vi "CSV reader.vi"(9 "x":dbl, 10 "Array":string[](array[string]), 11 "Number CSV":dbl) -> ()   [LabVIEW 2014]
uses:
  <vilib>/Utility/file.llb/Read From Spreadsheet File (DBL).vi
panel:
  out "all rows":dbl[][](array[numeric]) format="%0.3f"
  in  "index (col)":i32
  out "Gripper":dbl
  out "Left Encoder":dbl
  out "Left Drive":dbl
  out "Auton Left Arm":dbl
  out "Right Drive":dbl
  out "Right Encoder":dbl
  out "Auton Right Arm":dbl
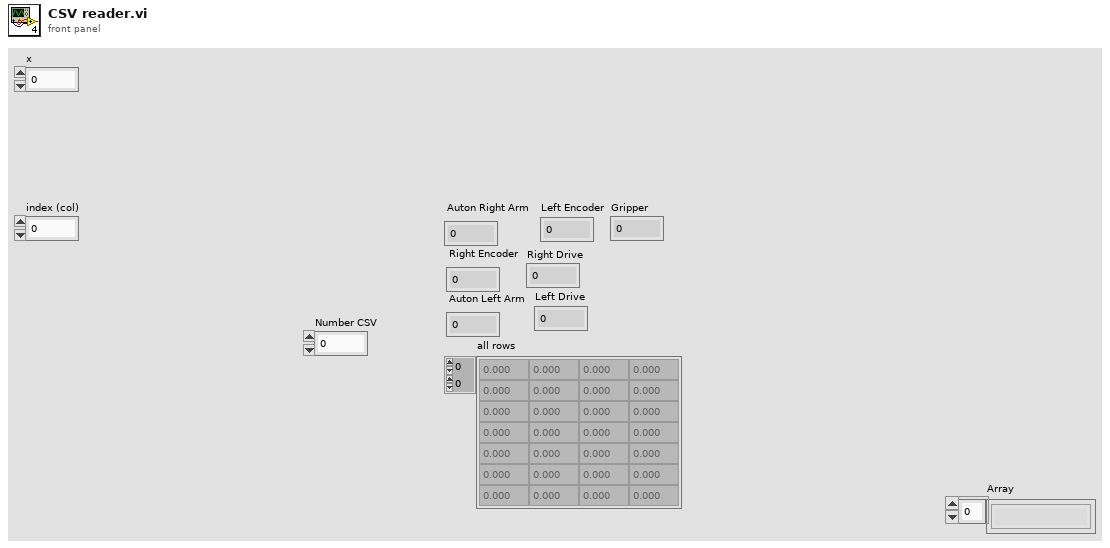
[diagram p1: front panel]
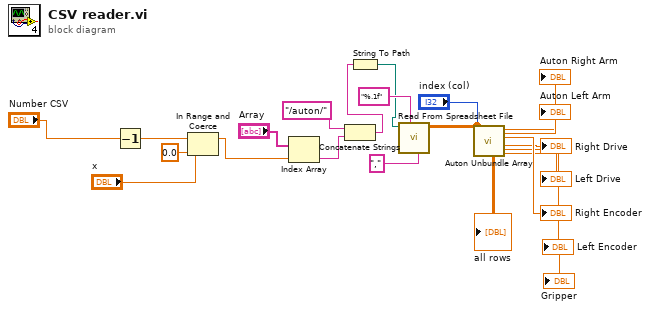
[diagram p0: block diagram]
diagram:
  n1 = Decrement(x="Number CSV") -> (x-1=w9:dbl)
  n2 = In Range and Coerce(upper limit=w9, x="x", lower limit=0.0) -> (coerced(x)=w6:dbl)  [unwired: 1 out]
  n3 = Index Array(array="Array", index=w6) -> (element=w4:string)
  n4 = Concatenate Strings("/auton/" ("string"), w4) -> (w2:string)
  n5 = String To Path(string=w2) -> (path=w1:path)
  n6 = call-poly <vilib>:"Read From Spreadsheet File.vi"("delimiter (\\t)"="," ("delimiter (\\t)"), "format (%.3f)"="%.1f", "file path (dialog if empty)"=w1) -> ("all rows"=w21:dbl[][])  [unwired: 4 in, 4 out]
  "all rows" <- w21
  n7 = call "Auton Unbundle Array.vi"("index (col)"="index (col)", "array"=w21) -> ("Left Drive"=→"Left Drive":dbl, "Right Drive"=→"Right Drive":dbl, "Right Encoder"=→"Right Encoder":dbl, "Auton Left Arm"=→"Auton Left Arm":dbl, "Left Encoder"=→"Left Encoder":dbl, "Auton Right Arm"=→"Auton Right Arm":dbl, "Gripper"=→"Gripper":dbl)  [unwired: 3 in]
